vi "Stop Core.vi"(10 "final error code":i32, 11 "Task_Abstr in":refnum<class "Task_Abstr.lvclass">) -> (3 "Task_Abstr out":refnum<class "Task_Abstr.lvclass">)   [LabVIEW 2025, in "Task_Abstr.lvlib" / "Task_Abstr.lvclass"]
doc: "<p>(<strong>Filename</strong>: <span class=\"dnl\">Actor Framework.lvlib:Actor.lvclass:Stop Core.vi</span>)</p>\n<p>Defines what the actor does before it stops. Use the <strong>final error code</strong> input to determine whether the actor shut down in response to an error.</p>\n<p>By default, this method passes the Stop message along to all <a href=\"nihelplauncher://docs/csh?context=lvcore_lvcomm_af_launch_nested_actor\">auto-stop nested actors</a>. A descendant class may override this method to define additional behavior, such as shutting down any processes the actor initiated in its override of the <a href=\"nihelplauncher://docs/csh?context=lvcore_lvcomm_af_actor_core\">Actor Core</a> method.</p>"
uses:
  Task_Abstr.lvclass
  <vilib>/ActorFramework/Time-Delayed Send Message/Time-Delay Override Options.ctl
  Task_Abstr.lvclass/Task_Abstr.ctl
  <vilib>/ActorFramework/Actor/Actor.lvclass
  <vilib>/ActorFramework/Actor Framework.lvlib
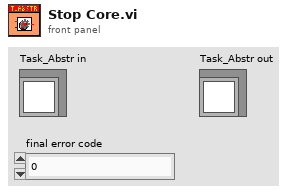
[diagram p1: front panel]
types:
  T1 = typedef "Actor Framework.lvlib/Time-Delay Override Options.ctl" = enum16{"Send next copy now", "Skip next scheduled copy", "Send next copy now and stop all further copies", "Stop all further copies"}
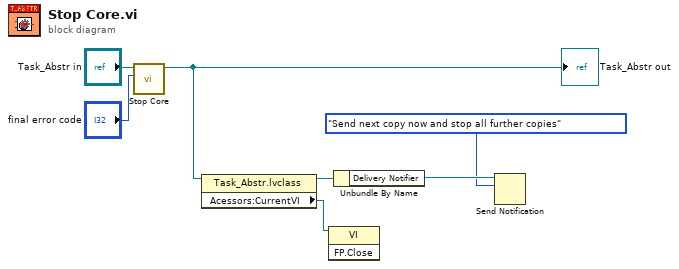
[diagram p0: block diagram]
diagram:
  n1 = call-parent "Stop Core.vi"("final error code"="final error code", "Actor in"="Task_Abstr in") -> ("Actor out"=w5:refnum<class "Task_Abstr.lvclass">)  [unwired: 9 in]
  "Task_Abstr out" <- w5
  n2 = property class="Task_Abstr.lvclass"(reference=w5) -> (reference out=w2:refnum<class "Task_Abstr.lvclass">, "Acessors:CurrentVI"=w1:refnum<vi>)  [unwired: 1 in, 1 out]
  n3 = invoke class="VI" method="FP.Close"(reference=w1) -> ()  [unwired: 2 in, 3 out]
  n4 = Unbundle By Name(w2) -> ("Delivery Notifier"=w4:refnum<notifier>)
  n5 = Send Notification(notification=Time-Delay_Override_Options."Send next copy now and stop all further copies", notifier=w4) -> ()  [unwired: 1 in, 2 out]
